vi "plotVariable.vi"() -> ()   [LabVIEW 2017]
uses:
  globalUtilities.vi
panel:
  in  "update interval":u32=5
  in  "stop":bool
  out "Waveform Chart":dbl(graph)
  in  "plot":bool
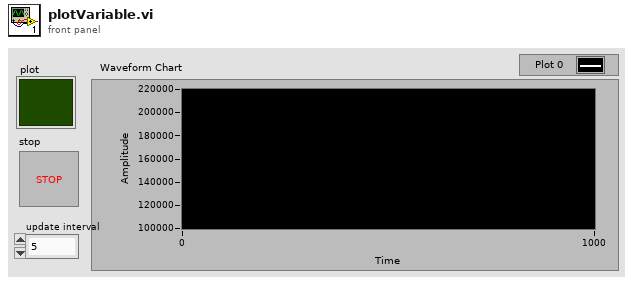
[diagram p1: front panel]
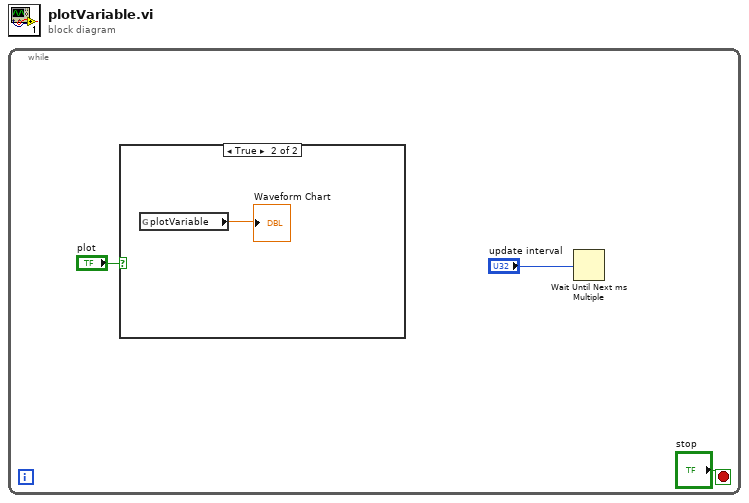
[diagram p0: block diagram]
diagram:
  n1 = while {
    stop <- "stop" stop-if-true
    n2 = case shown="True" "plot" {
      frame False {
      }
      frame True {
        n3 = global read "globalUtilities.vi" "plotVariable"() -> (→"Waveform Chart":dbl)
      }
    }
    n4 = Wait Until Next ms Multiple(millisecond multiple="update interval") -> ()  [unwired: 1 out]
  }
